vi "PAQmem_ReadAverage.vi"(8 "error in (no error)":errorcluster, 10 "ChunkDefinition":T2, 11 "PAQ-memory in":refnum<class "PAQ-memory.lvclass">) -> (0 "error out":errorcluster, 2 "Results":T1 {"status" format="%x"; "min" format="%.2f"; "max" format="%.2f"; "data" format="%.2f"}, 3 "PAQ-memory out":refnum<class "PAQ-memory.lvclass">)   [LabVIEW 2020, in "Sgraph_lib_V1.lvlib" / "PAQ-memory.lvclass"]
doc: "Read one Array of samples from a lower layer layer (higher resoltuion) and output the average and min/max results so they can be stored as one Higher Layer (lower resolution) element.\nOne sample containt and array of data elements."
uses:
  PAQ-memory.lvclass
  PAQ-memory.lvclass/PAQ-memory.ctl
  FAMM.lvclass
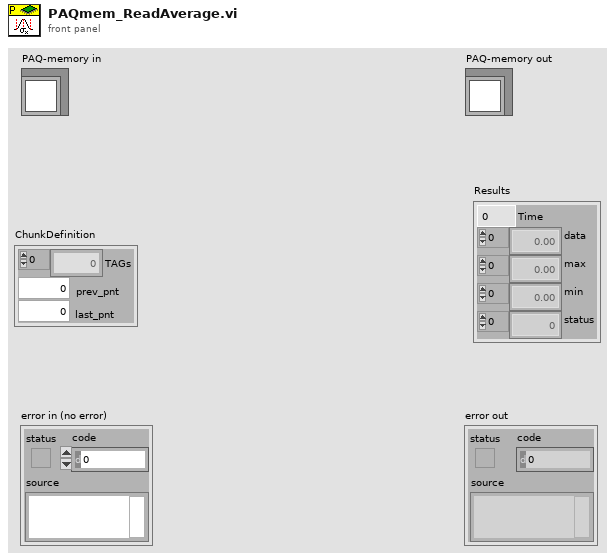
[diagram p1: front panel]
types:
  T1 = cluster{"Time":dbl, "data":dbl[], "max":dbl[], "min":dbl[], "status":u32[]}
  T2 = cluster{"TAGs":i32[], "prev_pnt":i32, "last_pnt":i32}
  T3 = cluster{"source":refnum<data-value>, "status":refnum<data-value>, "data":refnum<data-value>, "max":refnum<data-value>, "min":refnum<data-value>}[]
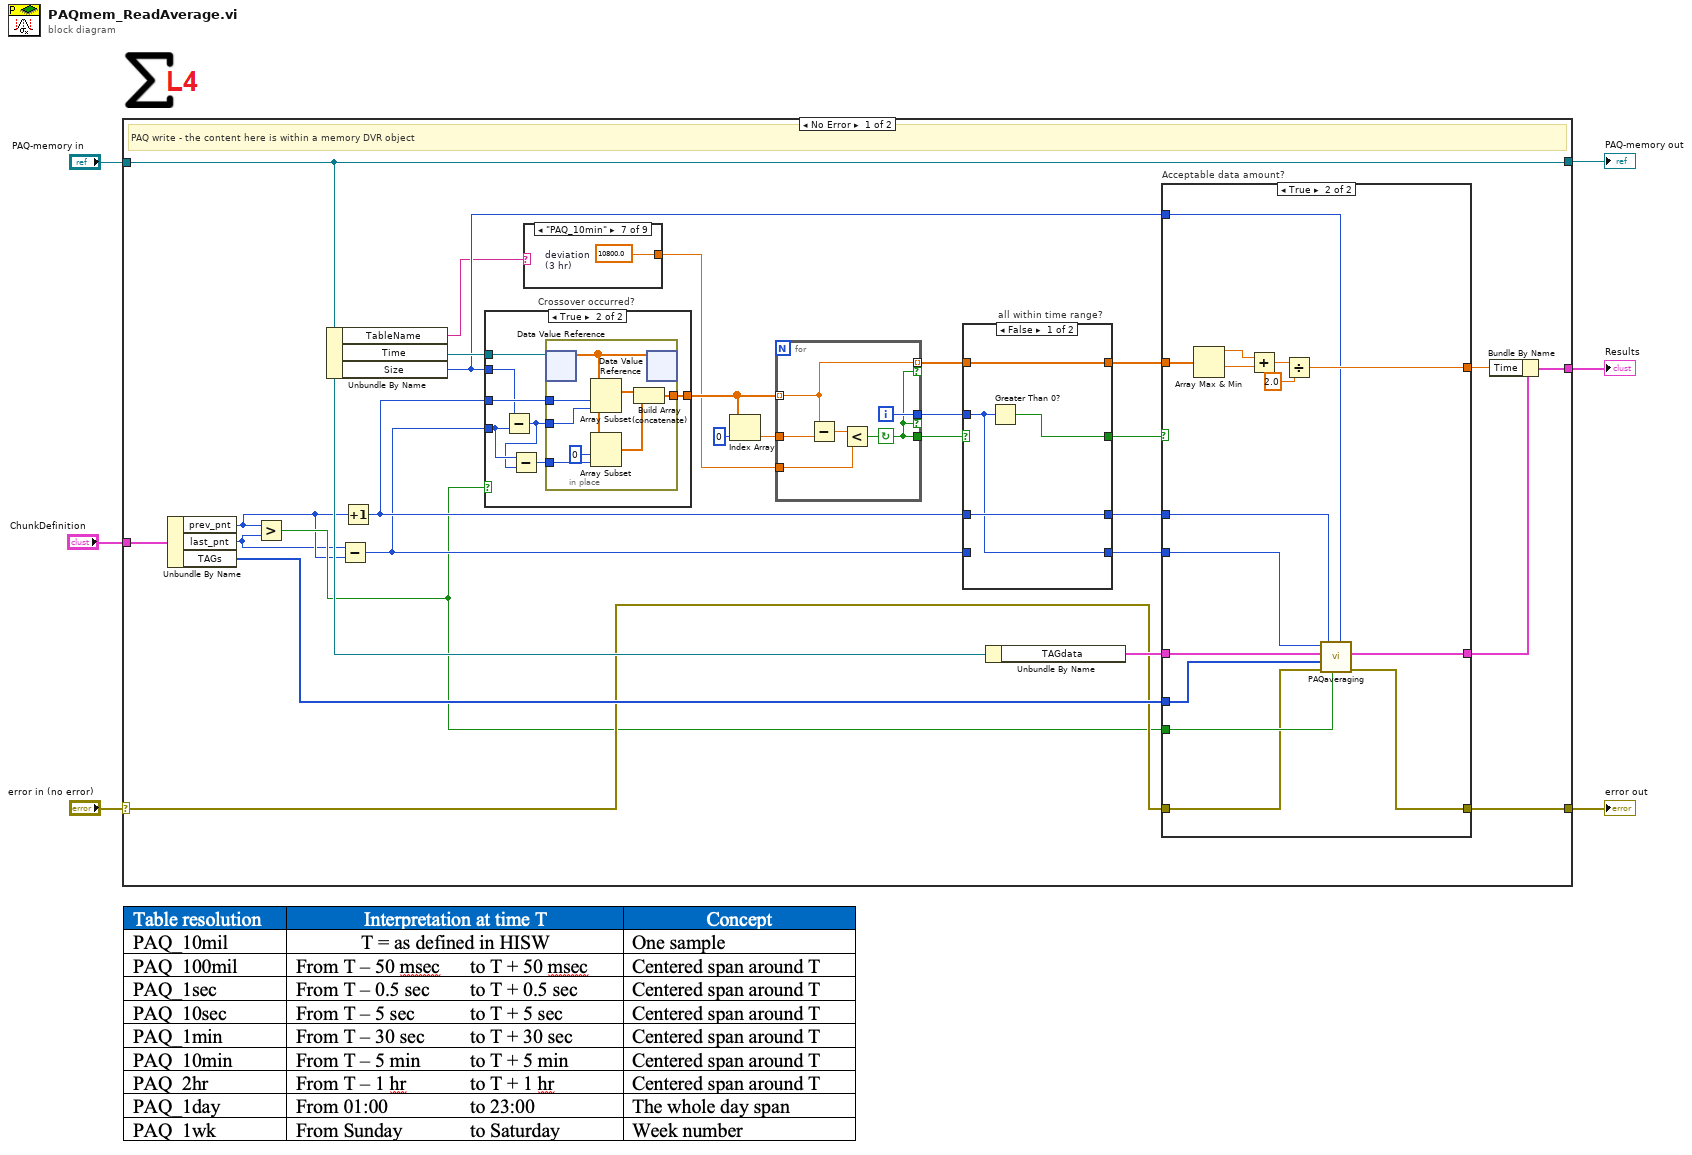
[diagram p0: block diagram]
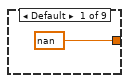
[diagram p3: hidden frame]
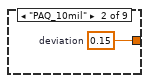
[diagram p4: hidden frame]
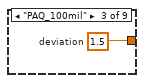
[diagram p5: hidden frame]
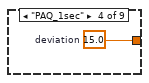
[diagram p6: hidden frame]
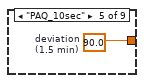
[diagram p7: hidden frame]
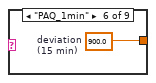
[diagram p8: hidden frame]
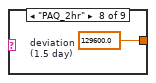
[diagram p9: hidden frame]
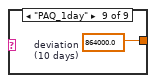
[diagram p10: hidden frame]
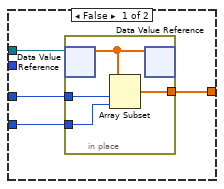
[diagram p11: hidden frame]
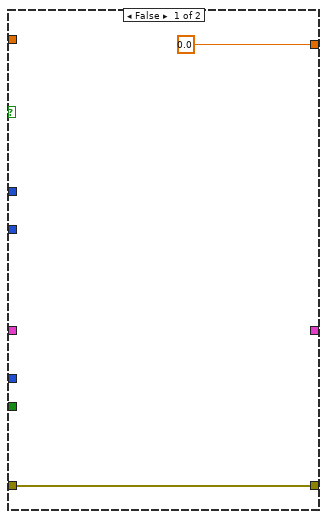
[diagram p12: hidden frame]
diagram:
  n1 = case shown="No Error" "error in (no error)" {
    selector: "error in (no error)" -> [w23 w99]
    tunnel: [w31 w99] -> w5
    tunnel: [w30 w98] -> w3
    tunnel: "PAQ-memory in" -> [w30 w98]
    tunnel: "ChunkDefinition" -> [w34 _]
    tunnel: [w32 _] -> w1
    frame No Error {
      # "PAQ write - the content here is within a memory DVR object"
      n2 = Unbundle By Name(w34) -> ("prev_pnt"=w15:i32, "last_pnt"=w14:i32, "TAGs"=w33:i32[])
      n3 = Greater?(x=w15, y=w14) -> (0:w16:bool)
      n4 = Unbundle By Name(w30) -> ("TableName"=w13:string, "Time"=w29:refnum<data-value>, "Size"=w22:i32)
      n5 = Subtract(x=w14, y=w15) -> (x-y=w18:i32)
      n6 = Increment(x=w15) -> (x+1=w19:i32)
      n7 = case "Crossover occurred?" shown="True" w16 {
        tunnel: w29 -> [w61 w72]
        tunnel: [w60 w66] -> w17
        tunnel: w19 -> [w59 w71]
        tunnel: w18 -> [w58 w68]
        tunnel: w22 -> [_ w70]
        frame False {
          n8 = in-place {
            in-place-border: w59 -> [w62]
            in-place-border: w58 -> [w64]
            in-place-border: [w63] -> w60
            n9 = in-place-dvr #1(w61) -> (w65:dbl[])  [unwired: 1 out]
            n10 = Array Subset(array=w65, index=w62, length=w64) -> (w63:dbl[])
            n11 = in-place-dvr #1(w65) -> ()  [unwired: 2 out]
          }
        }
        frame True {
          n12 = Subtract(x=w70, y=w68) -> (x-y=w67:i32)
          n13 = Subtract(x=w68, y=w67) -> (x-y=w69:i32)
          n14 = in-place {
            in-place-border: w71 -> [w80]
            in-place-border: w67 -> [w79]
            in-place-border: w69 -> [w76]
            in-place-border: [w73] -> w66
            n15 = in-place-dvr #2(w72) -> (w78:dbl[])  [unwired: 1 out]
            n16 = Array Subset(array=w78, index=w80, length=w79) -> (w75:dbl[])
            n17 = Array Subset(array=w78, index=0, length=w76) -> (w74:dbl[])
            n18 = Build Array (concatenate)(w75, w74) -> (w73:dbl[])
            n19 = in-place-dvr #2(w78) -> ()  [unwired: 2 out]
          }
        }
      }
      n20 = case shown="\"PAQ_10min\"" w13 {
        tunnel: [nan ("deviation\n(10 days)") w50 w51 w52 w53 w54 w55 w56 w57] -> w7
        frame Default {
        }
        frame "PAQ_10mil" {
          w50 = 0.15  # deviation
        }
        frame "PAQ_100mil" {
          w51 = 1.5  # deviation
        }
        frame "PAQ_1sec" {
          w52 = 15.0  # deviation
        }
        frame "PAQ_10sec" {
          w53 = 90.0  # deviation (1.5 min)
        }
        frame "PAQ_1min" {
          w54 = 900.0  # deviation (15 min)
        }
        frame "PAQ_10min" {
          w55 = 10800.0  # deviation (3 hr)
        }
        frame "PAQ_2hr" {
          w56 = 129600.0  # deviation (1.5 day)
        }
        frame "PAQ_1day" {
          w57 = 864000.0  # deviation (10 days)
        }
      }
      n21 = Index Array(array=w17, index=0) -> (element=w11:dbl)
      n22 = for {
        tunnel: w17 -> [w45] mode=indexing
        tunnel: w11 -> [w46]
        tunnel: [w47] -> w9 if=w44
        tunnel: [w44] -> w8
        tunnel: [w45] -> w10 mode=indexing if=w44
        tunnel: w7 -> [w43]
        i -> [w47]
        stop <- w44 continue-if-true
        n23 = Subtract(x=w45, y=w46) -> (x-y=w48:dbl)
        n24 = Less?(x=w48, y=w43) -> (x < y?=w44:bool)
      }
      n25 = case "all within time range?" shown="False" w8 {
        selector: w8 -> [_ w41]
        tunnel: w9 -> [w35 _]
        tunnel: w10 -> [w37 w42]
        tunnel: [w37 w42] -> w24
        tunnel: [w36 w41] -> w28
        tunnel: w19 -> [w38 w40]
        tunnel: [w38 w40] -> w26
        tunnel: w18 -> [_ w39]
        tunnel: [w35 w39] -> w25
        frame False {
          n26 = Greater Than 0?(x=w35) -> (x > 0?=w36:bool)
        }
        frame True {
        }
      }
      n27 = Unbundle By Name(w30) -> ("TAGdata"=w27:T3)
      n28 = case "Acceptable data amount?" shown="True" w28 {
        tunnel: w27 -> [_ w91]
        tunnel: w33 -> [_ w85]
        tunnel: w26 -> [_ w83]
        tunnel: w25 -> [_ w84]
        tunnel: w24 -> [_ w97]
        tunnel: w23 -> [w82 w89]
        tunnel: [w82 w88] -> w31
        tunnel: [0.0 w92] -> w20
        tunnel: w16 -> [_ w90]
        tunnel: w22 -> [_ w87]
        tunnel: [_ w86] -> w21
        frame False {
        }
        frame True {
          n29 = Array Max & Min(array=w97) -> (max value=w96:dbl, min value=w95:dbl)  [unwired: 2 out]
          n30 = Add(x=w96, y=w95) -> (x+y=w94:dbl)
          n31 = Divide(x=w94, y=2.0) -> (x/y=w92:dbl)
          n32 = call "PAQaveraging.vi"("Size"=w87, "Crossover?"=w90, "Index"=w83, "error in (no error)"=w89, "TAGs"=w85, "TAGdata"=w91, "Length"=w84) -> ("error out"=w88:errorcluster, "Results"=w86:T1)  [unwired: 3 in]
        }
      }
      n33 = Bundle By Name(cluster=w21, "Time"=w20) -> (w32:T1)
    }
    frame Error {
    }
  }
  "error out" <- w5
  "PAQ-memory out" <- w3
  "Results" <- w1
